vi "ContMotion.vi"(0 "Offset":i32, 5 "I/O chan for motion end":i32=2, 6 "steps between scans":sgl format="%.2f", 7 "1-D (F) 2-D (T)":bool, 8 "total steps in line":i32=100, 9 "Axis":i32=1 min=1 max=4, 10 "lines per scan":i32=128, 11 "I/O chan for motor pulse":i32=7) -> (3 "Output String":string)   [LabVIEW 2022 SP3]
uses:
  -MotionRoutines/MotionGlobals.vi
panel:
  in  "Direction line":i32=3
  out "length":i32
  # "Not used anymore"
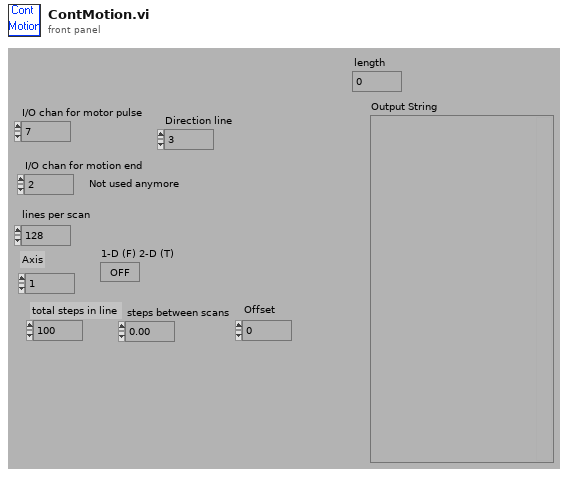
[diagram p1: front panel]
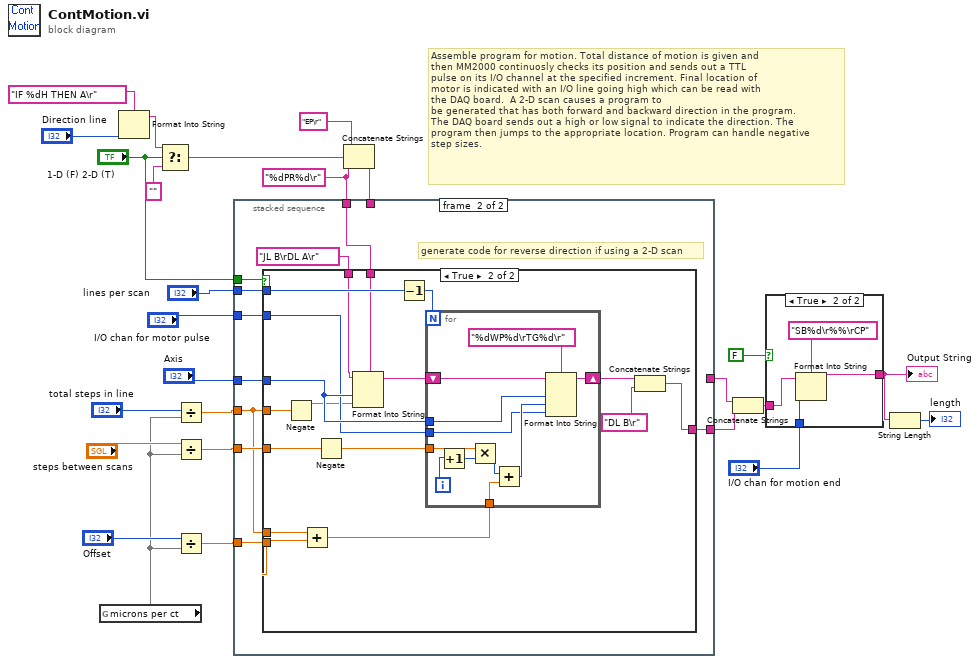
[diagram p0: block diagram]
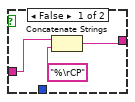
[diagram p2: hidden frame]
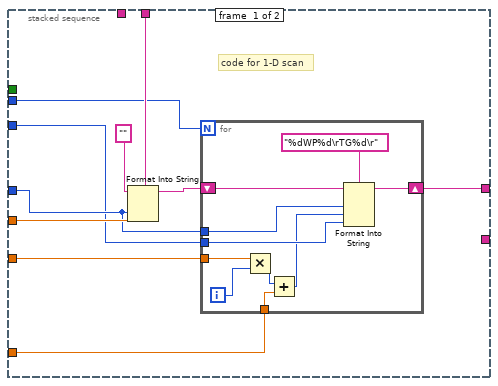
[diagram p3: hidden frame]
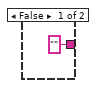
[diagram p4: hidden frame]
diagram:
  w17 = "%dPR%d\r"
  # "Assemble program for motion. Total distance of motion is given and\nthen MM2000 continuosly checks its position and sends out a TTL\npulse on its I/O channel at the specified increment. Final location of \nmotor is indicated with an I/O line going high which can be read with\nthe DAQ board.  A 2-D scan causes a program to \nbe generated that has both forward and backward direction in the program.\nThe DAQ board sends out a high or low signal to indicate the direction. The \nprogram then jumps to the appropriate location. Program can handle negative\nstep sizes."
  n1 = global read "MotionGlobals.vi" "microns per ct"() -> (w1)
  n2 = Format Into String(format string="IF %dH THEN A\r" ("f"), "Direction line") -> (resulting string=w10:string)  [unwired: 2 in, 1 out]
  n3 = Select(t=w10, s="1-D (F) 2-D (T)", f="") -> (s? t:f=w20:string)
  n4 = Divide(x="total steps in line", y=w1) -> (x/y=w6:dbl)
  n5 = Divide(x="steps between scans", y=w1) -> (x/y=w4:sgl)
  n6 = Divide(x="Offset", y=w1) -> (x/y=w3:dbl)
  n7 = Concatenate Strings("EP\r", w20, w17) -> (w19:string)
  n8 = stacked-sequence {
    tunnel: w19 -> [w36 _]
    tunnel: w6 -> [w33 w47]
    tunnel: w4 -> [w32 w56]
    tunnel: "lines per scan" -> [w27 w55]
    tunnel: w3 -> [w29 w54]
    tunnel: "Axis" -> [w31 w53]
    tunnel: [w30 _] -> w15
    tunnel: "I/O chan for motor pulse" -> [w28 w52]
    tunnel: "1-D (F) 2-D (T)" -> [_ w51]
    tunnel: w17 -> [_ w49]
    tunnel: [_ w48] -> w16
    frame #0 {
      # "code for 1-D scan"
      n9 = Format Into String(format string=w36, initial string="", w31, w33) -> (resulting string=w34:string)  [unwired: 1 in, 1 out]
      n10 = for {
        N: w27 -> [_]
        shift-right: [w45] -> w30
        shift-left: w34 -> [w44]
        tunnel: w29 -> [w43]
        tunnel: w32 -> [w41]
        tunnel: w31 -> [w40]
        tunnel: w28 -> [w39]
        i -> [w37]
        n11 = Multiply(x=w41, y=w37) -> (x*y=w42:i32)
        n12 = Add(x=w42, y=w43) -> (x+y=w38:i32)
        n13 = Format Into String(format string="%dWP%d\rTG%d\r", initial string=w44, w40, w38, w39) -> (resulting string=w45:string)  [unwired: 1 in, 1 out]
      }
    }
    frame #1 {
      # "generate code for reverse direction if using a 2-D scan"
      n14 = case shown="True" w51 {
        tunnel: w47 -> [_ w72]
        tunnel: w56 -> [_ w71]
        tunnel: w47 -> [_ w70]
        tunnel: w55 -> [_ w69]
        tunnel: w54 -> [_ w59]
        tunnel: w53 -> [_ w68]
        tunnel: w52 -> [_ w67]
        tunnel: w49 -> [_ w66]
        tunnel: "JL B\rDL A\r" ("Substring") -> [_ w65]
        tunnel: ["" w62] -> w48
        frame False {
        }
        frame True {
          n15 = Negate(x=w72) -> (-x=w61:dbl)
          n16 = Add(x=w70, y=w59) -> (x+y=w58:dbl)
          n17 = Negate(x=w71) -> (-x=w60:sgl)
          n18 = Format Into String(format string=w66, initial string=w65, w68, w61) -> (resulting string=w73:string)  [unwired: 1 in, 1 out]
          n19 = Decrement(x=w69) -> (x-1=w74:i32)
          n20 = for {
            N: w74 -> [_]
            shift-right: [w84] -> w64
            shift-left: w73 -> [w83]
            tunnel: w58 -> [w82]
            tunnel: w60 -> [w78]
            tunnel: w68 -> [w77]
            tunnel: w67 -> [w75]
            i -> [w79]
            n21 = Increment(x=w79) -> (x+1=w80:i32)
            n22 = Multiply(x=w78, y=w80) -> (x*y=w81:i32)
            n23 = Add(x=w81, y=w82) -> (x+y=w76:i32)
            n24 = Format Into String(format string="%dWP%d\rTG%d\r", initial string=w83, w77, w76, w75) -> (resulting string=w84:string)  [unwired: 1 in, 1 out]
          }
          n25 = Concatenate Strings(w64, "DL B\r" ("Substring")) -> (w62:string)
        }
      }
    }
  }
  n26 = Concatenate Strings(w15, w16) -> (w14:string)
  n27 = case shown="True" FALSE ("Case Constant\n(See Context Help)") {
    tunnel: [w86 w92] -> w23
    tunnel: w14 -> [w88 w90]
    tunnel: "I/O chan for motion end" -> [_ w89]
    frame False {
      n28 = Concatenate Strings(w88, "%\rCP") -> (w86:string)
    }
    frame True {
      n29 = Format Into String(format string="SB%d\r%%\rCP", initial string=w90, w89) -> (resulting string=w92:string)  [unwired: 1 in, 1 out]
    }
  }
  "Output String" <- w23
  n30 = String Length(string=w23) -> (length=→"length":i32)
